vi "UpdateDOUIcontrol.vi"(8 "error in (no error)":errorcluster, 9 "String":string, 10 "Value":bool, 11 "Data Value Reference in":T1) -> (0 "error out":errorcluster, 3 "Data Value Reference out":T1)   [LabVIEW 2022 SP3, in "TopLevel.lvclass"]
uses:
  TopLevel.lvclass
  <vilib>/TELLC/Dynamic CVT API/TD Dynamic CVT DVR--ref.ctl
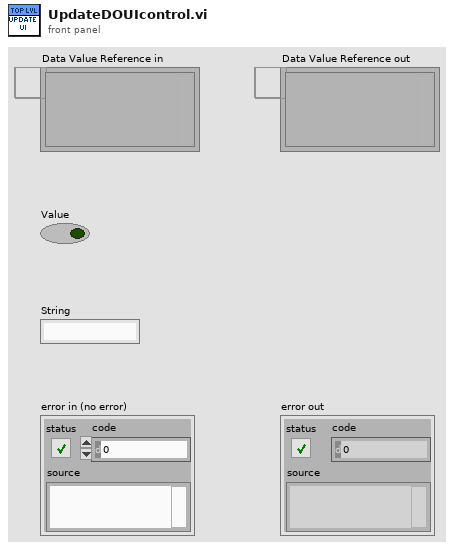
[diagram p1: front panel]
types:
  T1 = typedef "TD Dynamic CVT DVR--ref.ctl" = refnum<data-value>
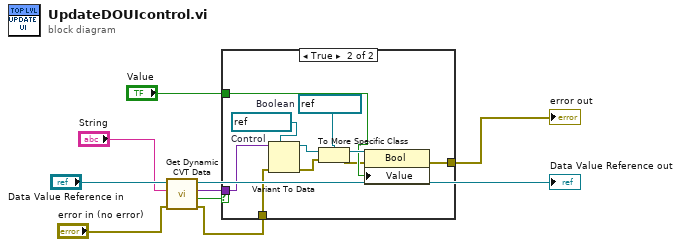
[diagram p0: block diagram]
diagram:
  n1 = call <vilib>:"Get Dynamic CVT Data.vi"("error in (no error)"="error in (no error)", "DataName"="String", "dCVT DVR"="Data Value Reference in") -> ("error out"=w6:errorcluster, "found"=w4:bool, "value"=w5:variant, "dCVT DVR out"=→"Data Value Reference out":T1)  [unwired: 5 in]
  n2 = case shown="True" w4 {
    tunnel: w5 -> [_ w20]
    tunnel: w6 -> [w10 w15]
    tunnel: "Value" -> [_ w13]
    tunnel: [w10 w11] -> w7
    frame False {
    }
    frame True {
      w18 = refnum<vi> refnum  # Boolean
      w19 = refnum<vi> refnum  # Control
      n3 = Variant To Data(error in=w15, type=w19, Variant=w20) -> (data=w17:refnum<vi>, error out=w16:errorcluster)
      n4 = To More Specific Class(target class=w18, reference=w17, error in=w16) -> (specific class reference=w14:refnum<vi>, error out=w12:errorcluster)
      n5 = property class="Bool"(reference=w14, error in=w12, "Value"=w13) -> (error out=w11:errorcluster)  [unwired: 1 out]
    }
  }
  "error out" <- w7
